vi "User Select From List.vi"(7 "list values":string[](array[string]), 8 "error in":errorcluster, 9 "timeout (s)":dbl=300.0, 10 "default index(0)":i32, 11 "prompt":string) -> (0 "error out":errorcluster, 1 "cancelled?":bool, 2 "string out":string, 3 "index out":i32, 4 "timeout?":bool)   [LabVIEW 2012]
panel:
  out "prompt display":string
  in  "user input":i32(ring) items=["Crossfire", "Typhon", "Krypton"]
  in  "cancel btn":bool
  in  "OK btn":bool
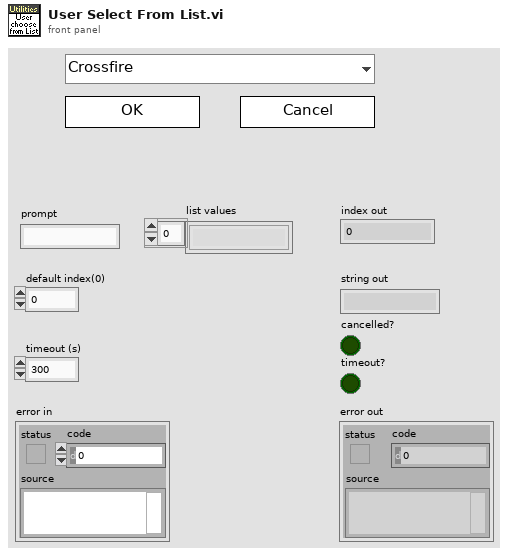
[diagram p1: front panel]
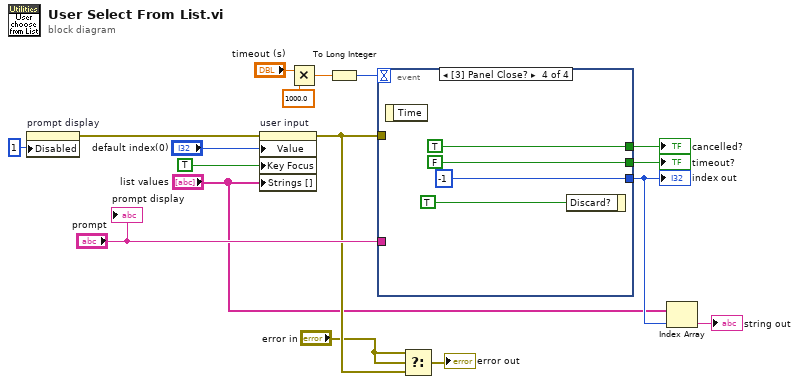
[diagram p0: block diagram]
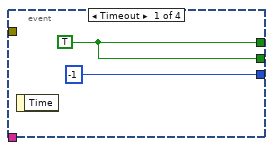
[diagram p2: hidden frame]
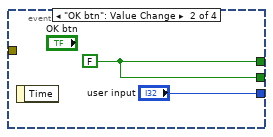
[diagram p3: hidden frame]
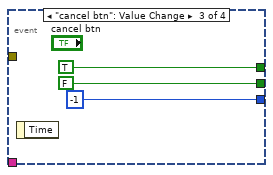
[diagram p4: hidden frame]
diagram:
  n1 = property on="prompt display" class="Str"("Disabled"=u8 1) -> (error out=w4:errorcluster)  [unwired: 2 in, 1 out]
  n2 = property on="user input" class="Ring (strict)"(error in=w4, "Value"="default index(0)", "Key Focus"=TRUE, "Strings []"="list values") -> (error out=w7:errorcluster)  [unwired: 1 in, 1 out]
  n3 = Multiply(x="timeout (s)", y=1000.0) -> (x*y=w13:dbl)
  n4 = To Long Integer(number=w13) -> (32bit integer=w14:i32)
  n5 = event shown="[3] Panel Close?" {
    selector: _ -> [_ _ _ _]
    dyn-events: _ -> [_ _ _ _]
    timeout: w14 -> [_ _ _ _]
    tunnel: w7 -> [_ _ _ _]
    tunnel: "prompt" -> [_ _ _ _]
    tunnel: [w19 w21 TRUE TRUE] -> w9
    tunnel: [w19 w21 FALSE FALSE] -> w8
    tunnel: [-1 ("user input") "user input" -1 ("user input") -1 ("user input")] -> w17
    event Timeout {
      w19 = TRUE
      n6 = event-data() -> ()  [unwired: 2 out]
    }
    event "OK btn": Value Change {
      w21 = FALSE
      n7 = event-data() -> ()  [unwired: 2 out]
    }
    event "cancel btn": Value Change {
      n8 = event-data() -> ()  [unwired: 2 out]
    }
    event Panel Close? {
      n9 = event-data() -> ()  [unwired: 2 out]
      n10 = event-data("Discard?"=TRUE) -> ()  [unwired: 1 in, 1 out]
    }
  }
  "index out" <- w17
  "cancelled?" <- w9
  "timeout?" <- w8
  n11 = Select(t="error in", s="error in", f=w7) -> (s? t:f=→"error out":errorcluster)
  n12 = Index Array(array="list values", index=w17) -> (element=→"string out":string)
  "prompt display" <- "prompt"
